vi "机器视觉图像采集.vi"() -> ()   [LabVIEW 2018]
uses:
  <vilib>/userdefined/High Color/IMAQdx.ctl
  <vilib>/vision/driver/NI_Vision_Acquisition_Software.lvlib
panel:
  out "Image":T1(plugin-control)
  in  "取消按钮":bool
  in  "IMAQdx Session":T2
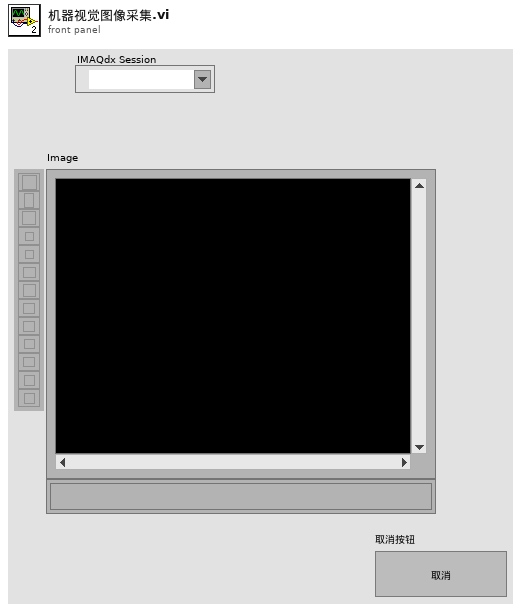
[diagram p1: front panel]
types:
  T1 = typedef "IMAQ Image.ctl" = refnum<image>
  T2 = typedef "IMAQdx.ctl" = refnum<k21>
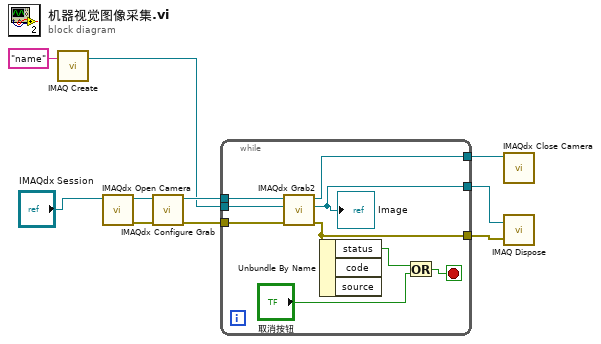
[diagram p0: block diagram]
diagram:
  n1 = call "IMAQ Create"("Image Name"="name") -> ("New Image"=w6:T1)  [unwired: 4 in, 1 out]
  n2 = call <vilib>:"IMAQdx Open Camera.vi"("Session In"="IMAQdx Session") -> ("error out"=w5:errorcluster, "Session Out"=w8:T2)  [unwired: 9 in]
  n3 = call <vilib>:"IMAQdx Configure Grab.vi"("error in"=w5, "Session In"=w8) -> ("error out"=w4:errorcluster, "Session Out"=w9:T2)  [unwired: 8 in]
  n4 = while {
    tunnel: w9 -> [w19]
    tunnel: w6 -> [w18]
    tunnel: w4 -> [w17]
    tunnel: [w13] -> w3
    tunnel: [w12] -> w2
    tunnel: [w11] -> w1
    stop <- w16 stop-if-true
    n5 = call <vilib>:"IMAQdx Grab2.vi"("error in"=w17, "Image In"=w18, "Session In"=w19) -> ("error out"=w12:errorcluster, "Image Out"=w11:T1, "Session Out"=w13:T2)  [unwired: 5 in, 1 out]
    "Image" <- w11
    n6 = Unbundle By Name(w12) -> ("status"=w15:bool)  [unwired: 2 out]
    n7 = Or(x=w15, y="取消按钮") -> (x .or. y?=w16:bool)
  }
  n8 = call <vilib>:"IMAQdx Close Camera.vi"("Session In"=w3) -> ()  [unwired: 10 in, 1 out]
  n9 = call "IMAQ Dispose"("Image"=w1, "error in (no error)"=w2) -> ()  [unwired: 4 in, 1 out]
